vi "Switch1.vi"() -> ()   [LabVIEW 2017]
panel:
  in  "Switch 1":bool
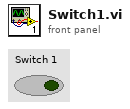
[diagram p1: front panel]
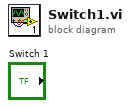
[diagram p0: block diagram]
diagram:
